vi "Create Buffers.vi"(7 "framework configuration":T1, 8 "error in (no error)":errorcluster, 11 "Framework in":refnum<class "Framework.lvclass">) -> (0 "error out":errorcluster, 3 "Framework out":refnum<class "Framework.lvclass">)   [LabVIEW 2017, in "DSF Core.lvlib" / "Framework.lvclass"]
uses:
  Framework.lvclass
  Typedefs/DSF Engine Framework Configuration.ctl
  Typedefs/DSF Engine Plugin Configuration.ctl
  Typedefs/DSF Timing Info.ctl
  Typedefs/DSF Engine Plugin Thread Configuration.ctl
  Typedefs/DSF Settings Info.ctl
  Typedefs/DSF Engine Transfer Group Configuration.ctl
  Typedefs/DSF Direction.ctl
  Typedefs/DSF Engine Transfer Configuration.ctl
  Typedefs/DSF Byte Order.ctl
  Typedefs/DSF Engine Channel Configuration.ctl
  Typedefs/DSF Data Type.ctl
  Buffer/Buffer.lvclass
  C:/Program Files (x86)/National Instruments/LabVIEW 2017/vi.lib/NI/Memory Manager/Classes/Pointer/Pointer.lvclass
  Framework.lvclass/Framework.ctl
  <vilib>/NI/Memory Manager/Classes/Pointer/Pointer.lvclass/Pointer.ctl
  Buffer/Buffer.lvclass/Buffer.ctl
  <vilib>/NI/Memory Manager/Classes/Pointer/Set Size.vi
  <vilib>/NI/Memory Manager/Classes/Pointer/Set Address.vi
  <vilib>/NI/Memory Manager/Classes/Pointer/Check Null Pointer.vi
  <vilib>/NI/Memory Manager/Classes/Pointer/Set Internal.vi
  <vilib>/NI/Memory Manager/Classes/Pointer/Errors.vi
  <vilib>/NI/Memory Manager/Classes/Pointer/Null Pointer.vi
  <vilib>/NI/Memory Manager/Classes/Pointer/Is Null.vi
  <vilib>/NI/Memory Manager/Classes/Pointer/Create Error.vi
  <vilib>/NI/Memory Manager/Classes/Pointer/Get Address.vi
  <vilib>/NI/Memory Manager/VIs/New Error Cluster Constant.vi
  <vilib>/NI/Memory Manager/VIs/New Error Cluster Constant (512B).vi
  <vilib>/NI/Memory Manager/VIs/Error Cluster.Set Status.vi
  <vilib>/NI/Memory Manager/VIs/Error Cluster.Set Code.vi
  <vilib>/NI/Memory Manager/VIs/Error Cluster.Set VI Source.vi
  <vilib>/NI/Memory Manager/Constants/Constants.vi
  <vilib>/NI/Memory Manager/Constants/Library Name.vi
  <vilib>/NI/Memory Manager/Classes/Pointer/Pointer Error Info.vi
  <vilib>/NI/Memory Manager/VIs/Source.Write.String.vi
  <vilib>/NI/Memory Manager/Constants/Pointer Class Name.vi
  Configuration/Required Buffer Size (Framework).vi
  Buffer/Buffers.lvclass
  DSF Core.lvlib
  <vilib>/NI/Memory Manager/Classes/Pointer/Pointer.lvclass
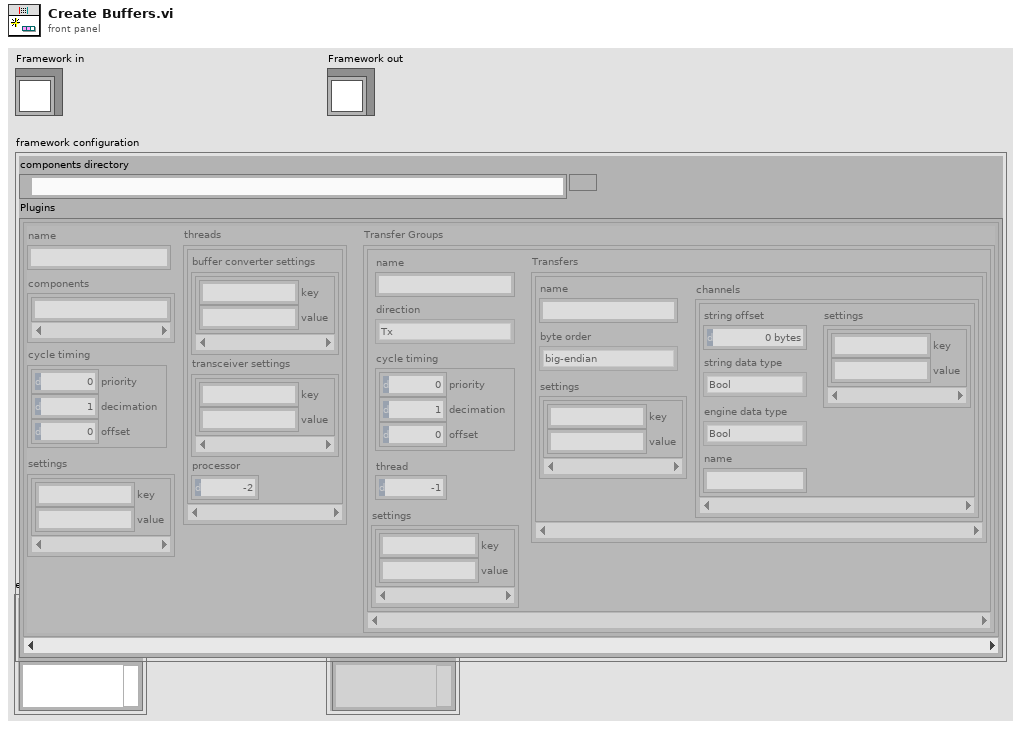
[diagram p1: front panel]
types:
  T1 = typedef "DSF Core.lvlib/DSF Engine Framework Configuration.ctl" = cluster{"components directory":path, "Plugins":T2[]}
  T2 = typedef "DSF Core.lvlib/DSF Engine Plugin Configuration.ctl" = cluster{"name":string, "components":string[], "cycle timing":T3, "threads":T4[], "Transfer Groups":T6[], "settings":T5}
  T3 = typedef "DSF Core.lvlib/DSF Timing Info.ctl" = cluster{"priority":u64, "decimation":u64, "offset":u64}
  T4 = typedef "DSF Core.lvlib/DSF Engine Plugin Thread Configuration.ctl" = cluster{"buffer converter settings":T5, "transceiver settings":T5, "processor":i32}
  T5 = typedef "DSF Core.lvlib/DSF Settings Info.ctl" = cluster{"key":string, "value":string}[]
  T6 = typedef "DSF Core.lvlib/DSF Engine Transfer Group Configuration.ctl" = cluster{"name":string, "direction":T7, "cycle timing":T3, "thread":i32, "settings":T5, "Transfers":T8[]}
  T7 = typedef "DSF Core.lvlib/DSF Direction.ctl" = enum8{"Tx", "Rx"}
  T8 = typedef "DSF Core.lvlib/DSF Engine Transfer Configuration.ctl" = cluster{"name":string, "byte order":T9, "settings":T5, "channels":T10[]}
  T9 = typedef "DSF Core.lvlib/DSF Byte Order.ctl" = enum8{"big-endian", "little-endian"}
  T10 = typedef "DSF Core.lvlib/DSF Engine Channel Configuration.ctl" = cluster{"string offset":u64, "string data type":T11, "engine data type":T11, "name":string, "settings":T5}
  T11 = typedef "DSF Core.lvlib/DSF Data Type.ctl" = enum8{"Bool", "SGL", "DBL", "I8", "I16", "I32", "I64", "U8", "U16", "U32", "U64"}
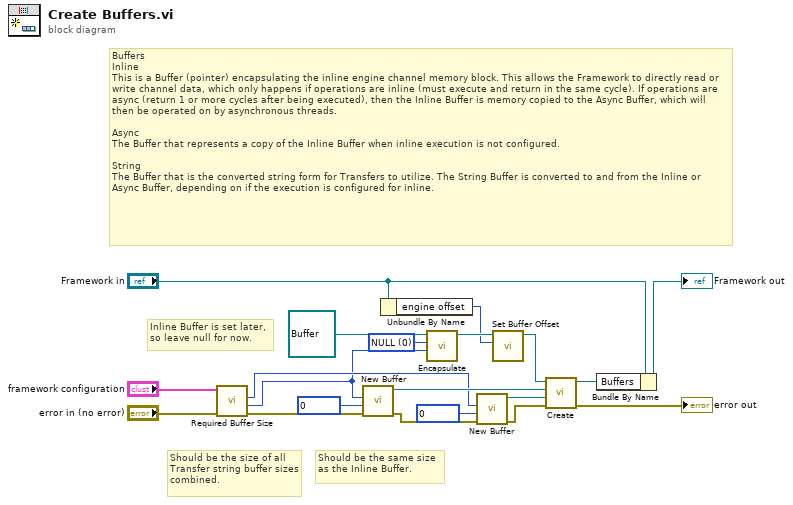
[diagram p0: block diagram]
diagram:
  w1 = u64 0 items=["NULL"] ("Null")
  # "Should be the size of all Transfer string buffer sizes combined."
  # "Should be the same size as the Inline Buffer."
  # "Buffers\nInline\nThis is a Buffer (pointer) encapsulating the inline engine channel memory block. This allows the Framework to directly read or write channel data, which only happens if operations are inline (must execute and return in the same cycle). If operations are async (return 1 or more cycles after being executed), then the Inline Buffer is memory copied to the Async Buffer, which will then be operated on by asynchronous threads.\n\nAsync\nThe Buffer that represents a copy of the Inline Buffer when inline execution is not configured.\n\nString\nThe Buffer that is the converted string form for Transfers to utilize. The String Buffer is converted to and from the Inline or Async Buffer, depending on if the execution is configured for inline."
  # "Inline Buffer is set later, so leave null for now."
  n1 = call-poly "Required Buffer Size.vi"("error in (no error)"="error in (no error)", "Framework Configuration in"="framework configuration") -> ("error out"=w14:errorcluster, "total engine buffer size"=w3:u64, "total string buffer size"=w8:u64)  [unwired: 6 in, 1 out]
  n2 = call "New Buffer.vi"("error in (no error)"=w14, "buffer offset"=u64 0, "buffer size"=w3) -> ("error out"=w17:errorcluster, "Buffer out"=w9:refnum<class "Buffer.lvclass">)  [unwired: 7 in]
  n3 = Unbundle By Name("Framework in") -> ("engine offset"=w2:u64)
  n4 = call <vilib>:"Encapsulate.vi"("size"=w3, "address"=w1, "Pointer in"=refnum<class "Buffer.lvclass"> refnum ("Inline Buffer (null)")) -> ("Pointer out"=w4:refnum<class "Buffer.lvclass">)  [unwired: 7 in, 1 out]
  n5 = call "New Buffer.vi"("error in (no error)"=w17, "buffer offset"=u64 0, "buffer size"=w8) -> ("error out"=w20:errorcluster, "Buffer out"=w16:refnum<class "Buffer.lvclass">)  [unwired: 7 in]
  n6 = call "Set Buffer Offset.vi"("buffer offset"=w2, "Buffer in"=w4) -> ("Buffer out"=w6:refnum<class "Buffer.lvclass">)  [unwired: 9 in]
  n7 = call "Create.vi"("error in (no error)"=w20, "String Buffer (null)"=w16, "Async Buffer (null)"=w9, "Inline Buffer (null)"=w6) -> ("error out"=→"error out":errorcluster, "Buffers out"=w19:refnum<class "Buffers.lvclass">)  [unwired: 6 in]
  n8 = Bundle By Name(cluster="Framework in", "Buffers"=w19) -> (→"Framework out":refnum<class "Framework.lvclass">)
